vi "GUI_kHz_Control_Center_beta.vi"() -> ()   [LabVIEW 2020]
uses:
  GUI_TestStand/Fire button.ctl
  Shared/GUI_Template/GUI_master/tcp_new_data_event.ctl
  Shared/GUI_Template/GUI_master/tcp new data cluster.ctl
  Device Drivers/DG645/subVIs/TriggerSource_TypDef.ctl
panel:
  in  "BASE PATH":path=path "Z:/software/control-all-loasis/kHzLPA/Developers Version"
  in  "stop":bool
  in  "Tab Control":enum32{"Devices", "Parameters"}(tab)=enum."Parameters"
  in  "GUIdevice 6":string="kHz_Zaber_Compressor"
  in  "GUIdevice 2":string="kHz_1Wire"
  in  "GUIdevice 1":string="kHz_Alicat"
  in  "GUIdevice 3":string="kHz_Hexapod_Target"
  in  "GUIdevice 4":string="kHz_DG645_ShotControl"
  in  "GUIdevice 5":string="kHz_Zaber_Compressor"
  out "error IO":errorcluster
  out "tcp data event":T1
  in  "fire::4":string="fire>>force" caption="fire text"
  in  "Step size":dbl=0.01 min=0.001 max=1.0 step=0.001 format="%.3f"
  in  "Rate (Hz)":dbl=0.3
  in  "Allow Fire Continues":bool
  out "Fire continues Indicator":bool caption="Fire continuous"
  in  "Trigger.Source::4":T2 caption="SRS Trigger Mode"
  in  "LVStarter":bool caption="PicoL GUI"
  in  "Scan":T3(ring)
  in  "<command>::3":bool caption="ABORT"
  in  "Position.Ch1::5":i32 caption="Ch1" min=0 max=250000 step=1
  in  "Google Drive":bool
  in  "MasterControl":bool caption="PicoL GUI"
  in  "GEECSplot":bool caption="PicoL GUI"
  in  "AddColumns":bool caption="PicoL GUI"
  in  "DB Editor":bool caption="PicoL GUI"
  in  "Exp Editor":bool caption="PicoL GUI"
  in  "kHz Interactive":bool caption="PicoL GUI"
  in  "RemoteDesktop":bool caption="PicoL GUI"
  in  "Search Log":bool caption="PicoL GUI"
  in  "New Google\nExpLog for new day?":bool=TRUE
  in  "LogEpilog":bool caption="LogTable"
  in  "Create Log":bool caption="LogTable"
  in  "Position.Channel 1::2":T4(ring) caption="XH1"
  in  "Position.Channel 2::2":T4(ring) caption="XH2"
  in  "Position.Channel 3::2":T4(ring) caption="XH3"
  in  "Position.Channel 4::2":T4(ring) caption="XH4"
  in  "Position.Channel 5::2":T4(ring) caption="d-scan wedge"
  in  "Position.Channel 6::2":T4(ring) caption="EC wedge"
  in  "Position.Channel 8::2":T4(ring) caption="ND6+"
  in  "Position.Channel 7::2":T4(ring) caption="ExitMode wedge"
  in  "Pressure.device 1::1":dbl=3.6 caption="Target Pressure" min=0.0 max=100.0
  in  "Pressure.device 2::1":dbl=10.0 caption="Fiber Pressure" min=-14.7 max=300.0
  in  "xpos::3":dbl=-18.95 caption="x" min=-22.5 max=22.5 step=0.1 format="%.3f"
  in  "zpos::3":dbl=-0.7 caption="z" min=-10.0 max=10.0 step=0.1 format="%.3f"
  in  "ypos::3":dbl=10.7 caption="y" min=-22.5 max=22.5 step=0.1 format="%.3f"
  in  "uangle::3":dbl caption="u" min=-7.5 max=7.5 step=0.1 format="%.3f"
  in  "vangle::3":dbl=0.0007 caption="v" min=-7.5 max=7.5 step=0.1 format="%.3f"
  in  "wangle::3":dbl=-0.0001 caption="w" min=-7.5 max=7.5 step=0.1 format="%.3f"
  in  "LogTable":bool
  in  "Fire Button":T5=TRUE
  in  "Jet trigger":bool caption="Jet Trigger"
  in  "Jet enable":bool caption="Jet Enable"
  in  "Set opening time (s)":dbl=0.004
  in  "Amplitude.Ch AB::4":dbl=4.0 caption="Amplitude Jet trigger" min=0.5 max=5.0 format="%.1f"
  in  "Delay.Ch B::4":dbl=0.004 caption="Opening time" min=-0.1 max=0.1 format="%#_6p"
  in  "value0:6":bool caption="Fire continues"
  in  "UDP error message":string
  # "kHz Control Center"
  # "Laser"
  # "1-wire flippers"
  # "\"+x\" is towards laser table\n\"+y\" is towards OAP\n\"+z\" is up"
  # "ABORT !"
  # "Tobi's LogMaker"
  # "Alicat"
  # "New\nScan\nTable"
  # "Compressor"
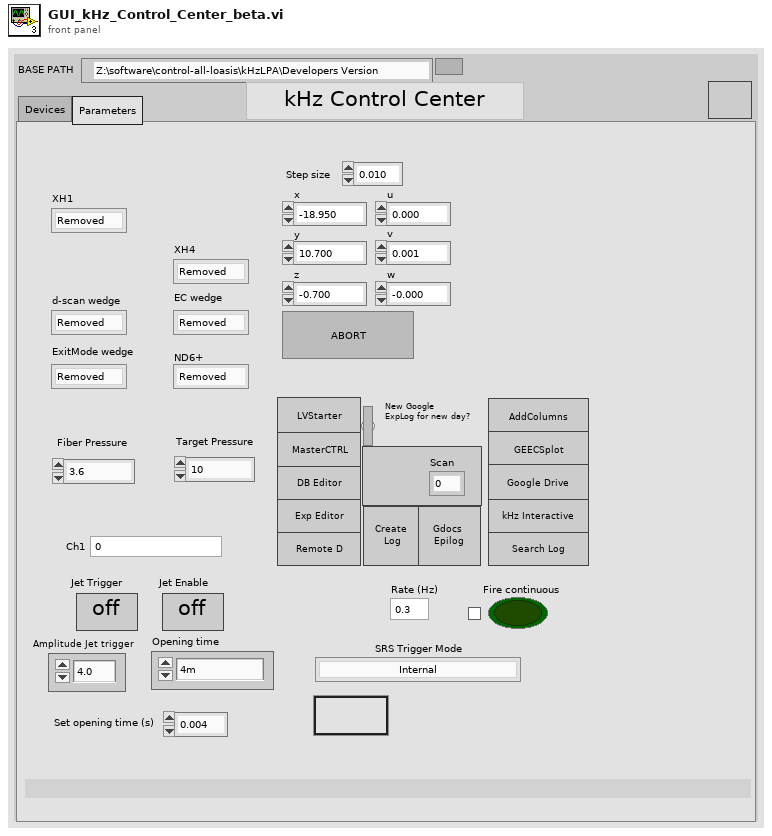
[diagram p1: front panel]
types:
  T1 = typedef "tcp_new_data_event.ctl" = refnum<user-event>
  T2 = typedef "TriggerSource_TypDef.ctl" = enum16{"Internal", "External rising edges", "External falling edges", "Single shot external rising edges", "Single shot external falling edges", "Single shot", "Line"}
  T3 = enum16{"0", "1", "2", "3", "4", "5", "6", "7", "8", "9", "10", "11", "12", "13", "14", "15", "16", "17", "18", "19", "20", "21", "22", "23", "24", "25", "26", "27", "28", "29", "30", "31", "32", "33", "34", "35", "36", "37", "38", "39", "40", "41", "42", "43", "44", "45", "46", "47", "48", "49", "50", "51", "52", "53", "54", "55", "56", "57", "58", "59", "60", "61", "62", "63", "64", "65", "66", "67", "68", "69", "70", "71", "72", "73", "74", "75", "76", "77", "78", "79", "81", "82", "83", "84", "85", "86", "87", "88", "89", "90", "91", "92", "93", "94", "95", "96", "97", "98", "99", ""}
  T4 = enum16{"Removed", "Inserted", "Unknown", "Moving"}
  T5 = typedef "Fire button.ctl" = bool
  T6 = typedef "tcp new data cluster.ctl" = cluster{"EventEnum":enum16{"new data", "connection status update"}, "Device name":string}
  T7 = enum32{"Invalid", "Standard", "Closed", "Hidden", "Minimized", "Maximized"}
  T8 = enum32{"invalid app kind", "Development System", "Run Time System", "Student Edition", "Embedded LabVIEW", "Evaluation", "Custom"}
  T9 = cluster{"Core":cluster{"Current VI Reference":refnum<vi>, "Close Panel on Exit?":bool}, "F":bool, "Jet trigger":bool, "Fire Continues Allowed":bool, "Tik1":u32}
  T10 = cluster{"Current VI Reference":refnum<vi>, "Close Panel on Exit?":bool}
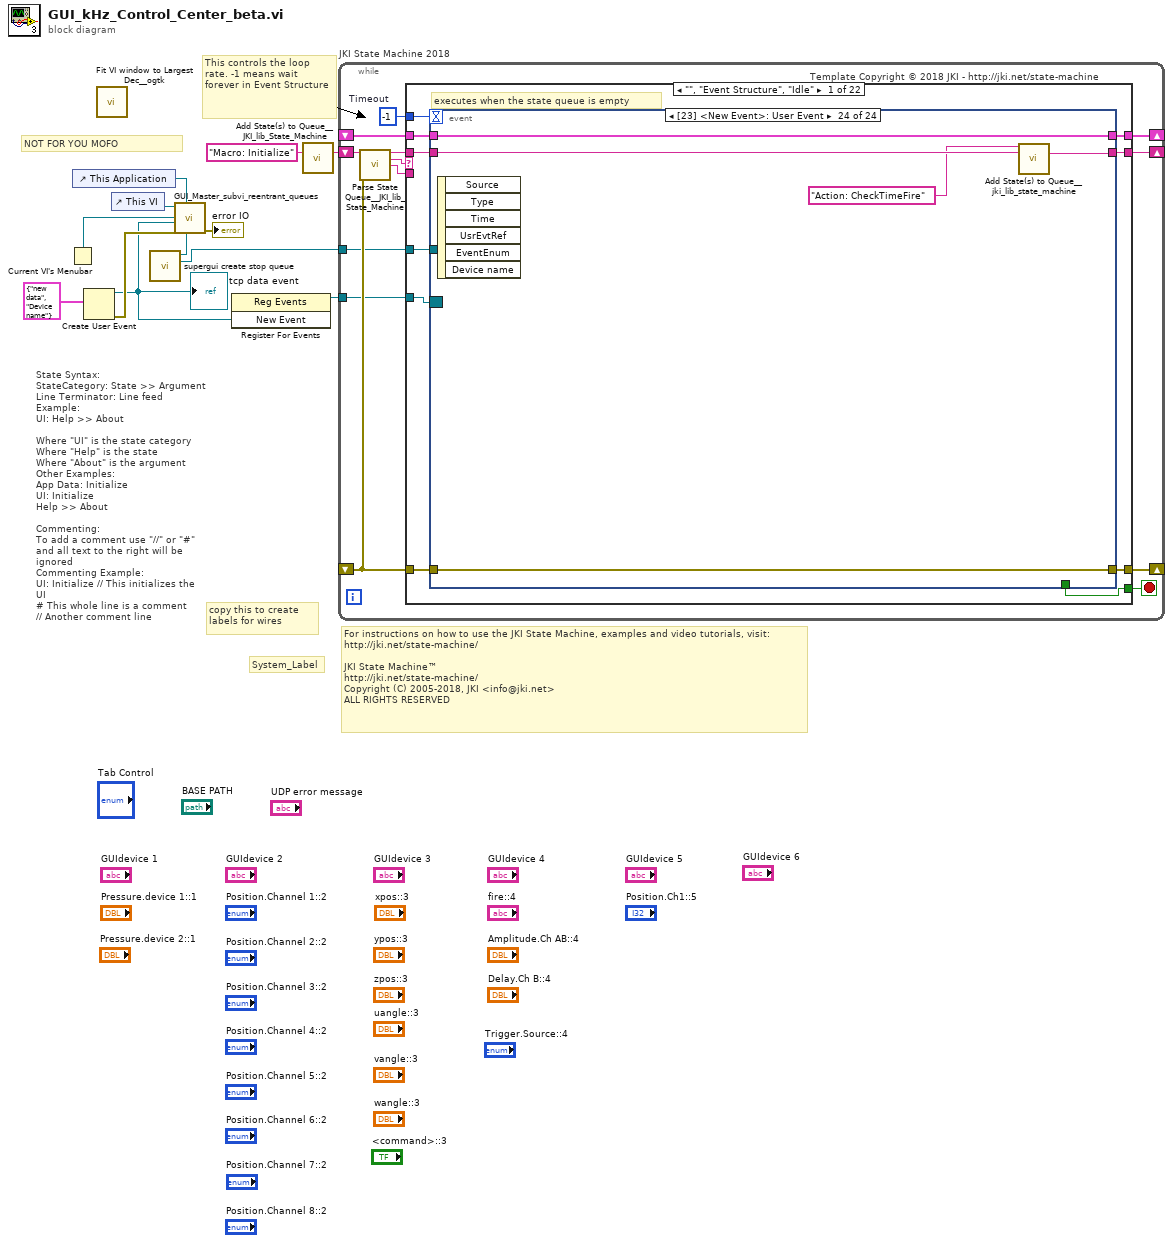
[diagram p0: block diagram]
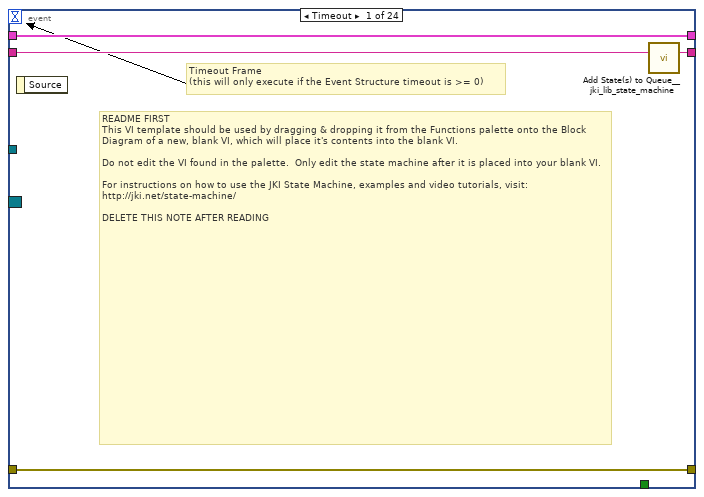
[diagram p2: hidden frame]
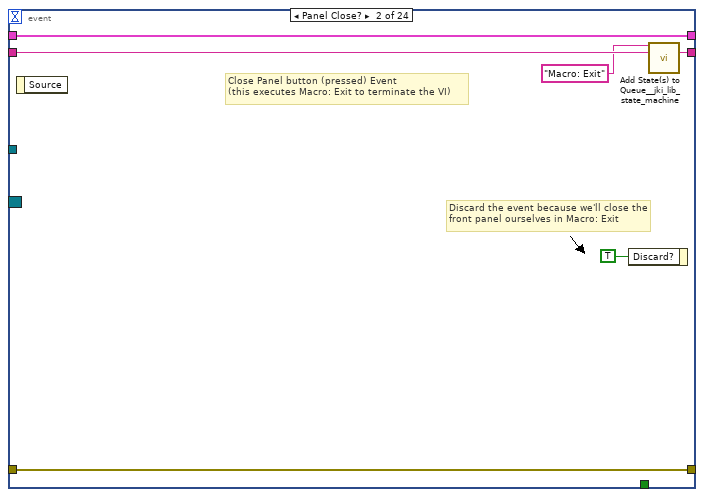
[diagram p3: hidden frame]
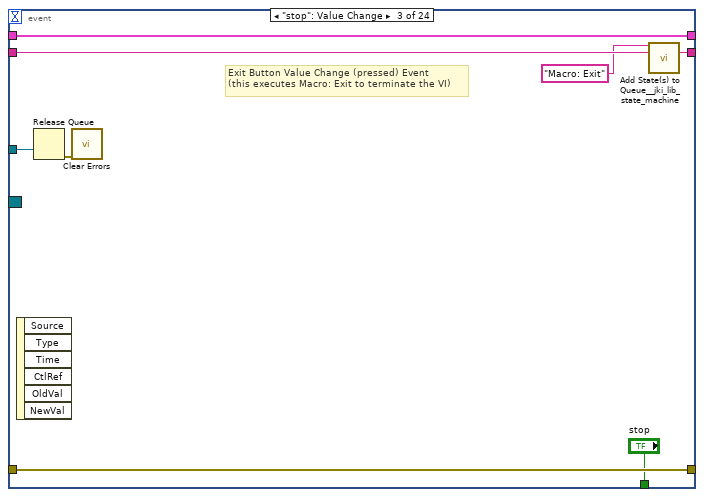
[diagram p4: hidden frame]
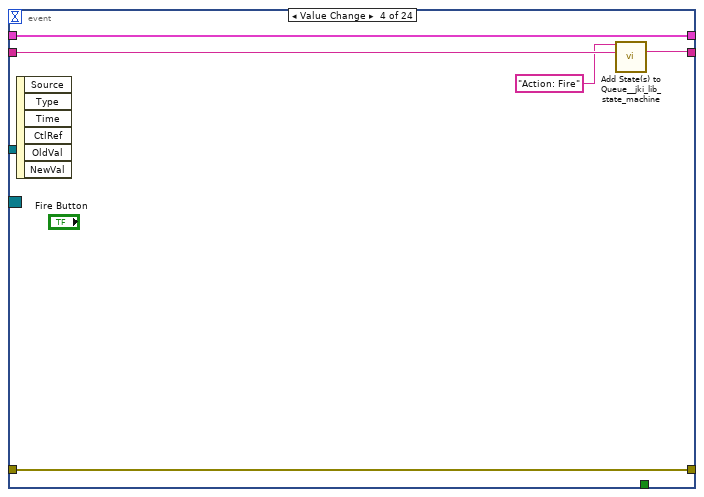
[diagram p5: hidden frame]
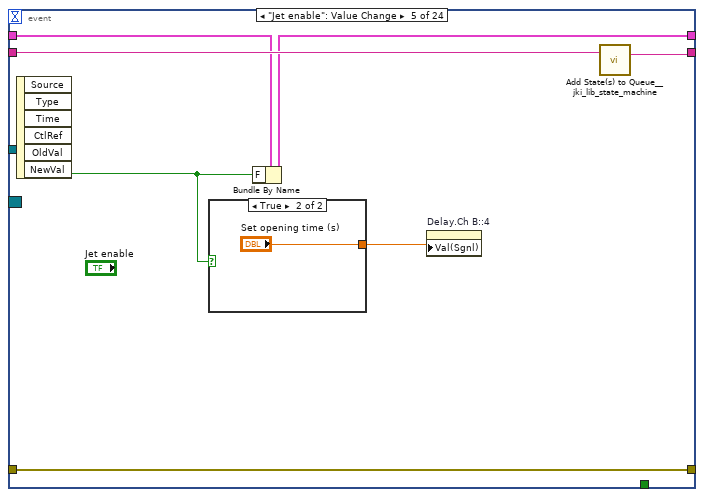
[diagram p6: hidden frame]
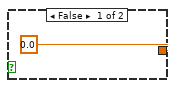
[diagram p7: hidden frame]
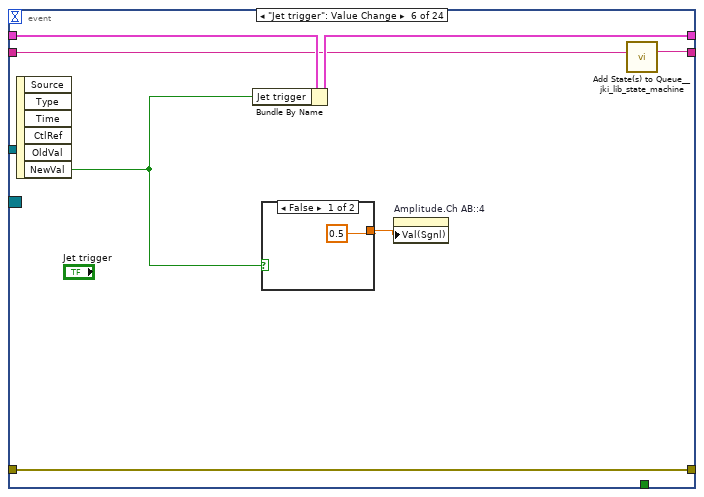
[diagram p8: hidden frame]
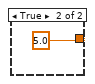
[diagram p9: hidden frame]
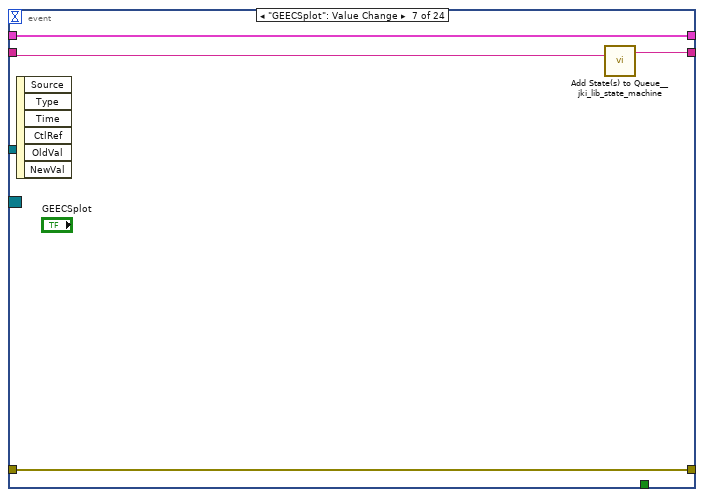
[diagram p10: hidden frame]
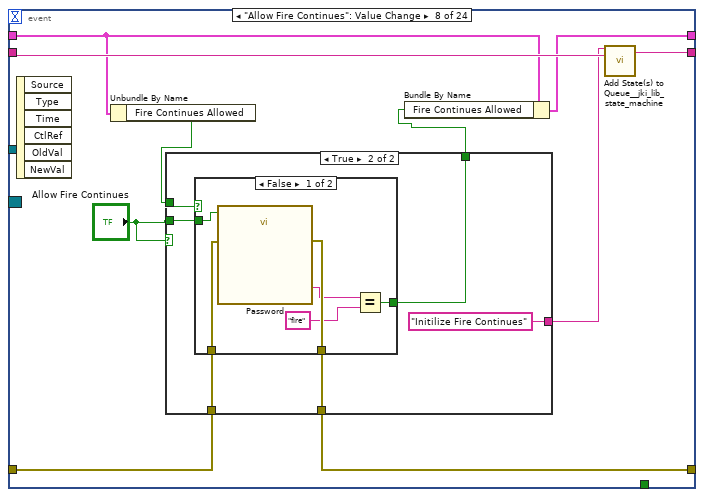
[diagram p11: hidden frame]
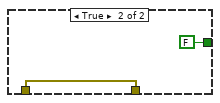
[diagram p13: hidden frame]
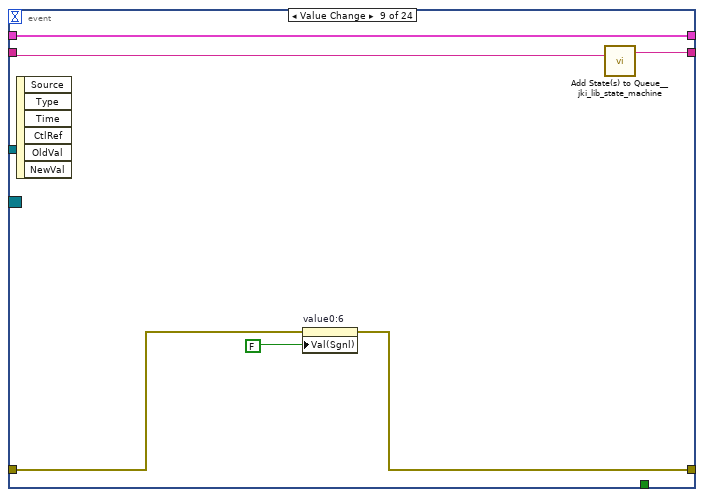
[diagram p14: hidden frame]
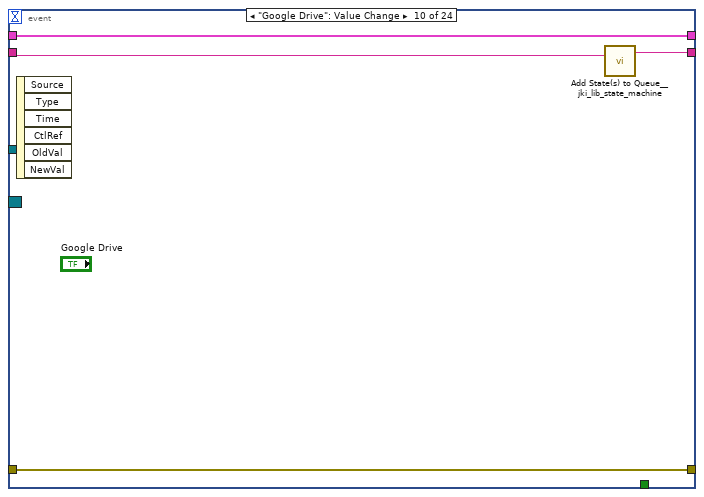
[diagram p15: hidden frame]
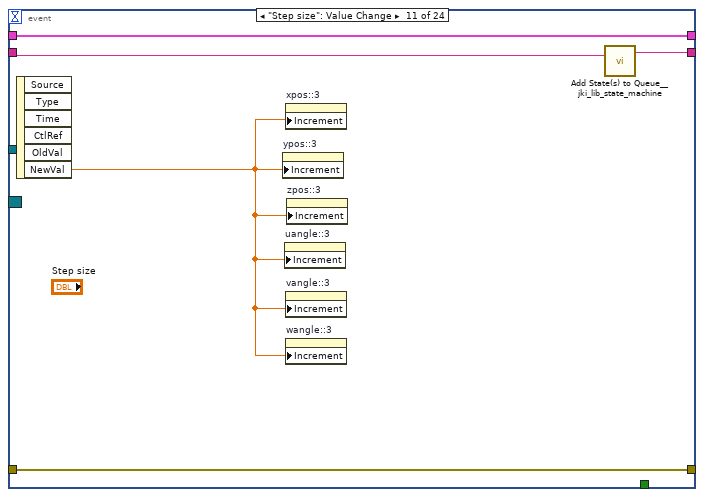
[diagram p16: hidden frame]
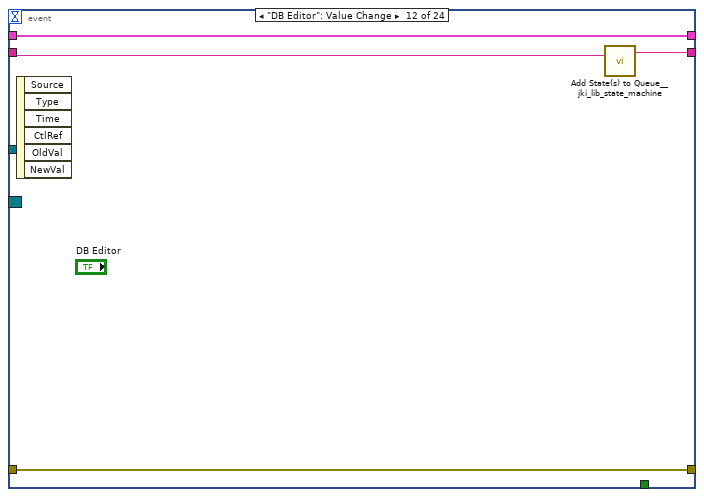
[diagram p17: hidden frame]
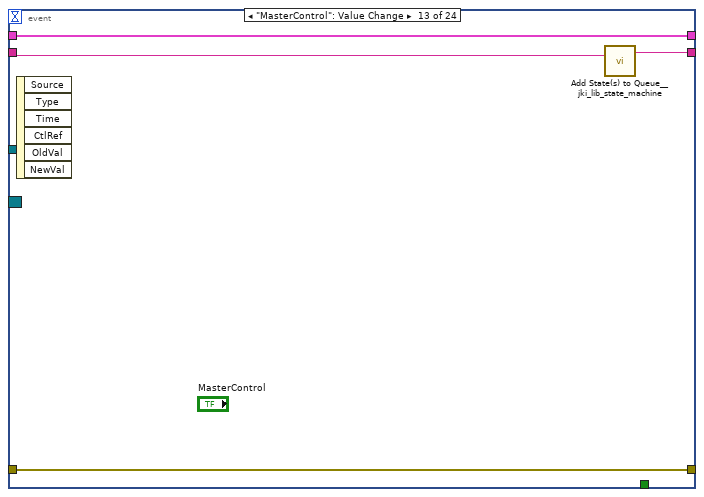
[diagram p18: hidden frame]
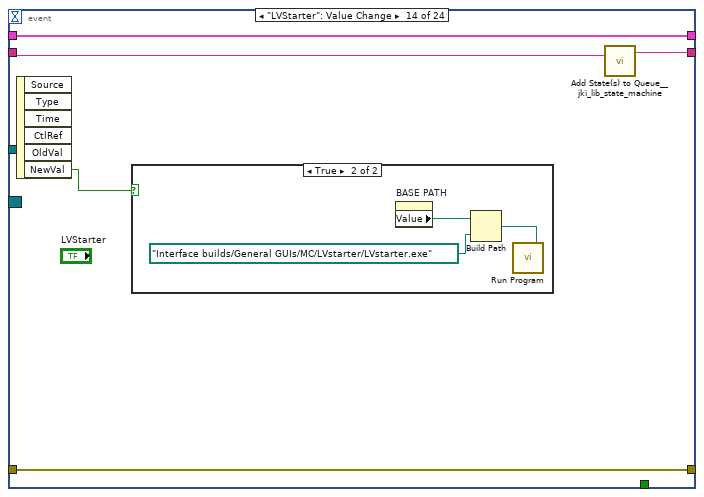
[diagram p19: hidden frame]
diagram:
  # "NOT FOR YOU MOFO"
  # "For instructions on how to use the JKI State Machine, examples and video tutorials, visit:\nhttp://jki.net/state-machine/\n\nJKI State Machine™\nhttp://jki.net/state-machine/\nCopyright (C) 2005-2018, JKI <info@jki.net>\nALL RIGHTS RESERVED"
  # "State Syntax:\nStateCategory: State >> Argument\nLine Terminator: Line feed\nExample:\nUI: Help >> About\n\nWhere \"UI\" is the state category\nWhere \"Help\" is the state\nWhere \"About\" is the argument\nOther Examples:\nApp Data: Initialize\nUI: Initialize\nHelp >> About\n\nCommenting:\nTo add a comment use \"//\" or \"#\" and all text to the right will be ignored\nCommenting Example:\nUI: Initialize // This initializes the UI\n# This whole line is a comment\n// Another comment line"
  # "copy this to create labels for wires"
  # "This controls the loop rate. -1 means wait forever in Event Structure"
  # "System_Label"
  n1 = Current VI's Menubar() -> (w6:refnum<k9>)
  n2 = control-ref of="This Application"() -> (w9:refnum<vi>)
  n3 = Create User Event(user event datatype=T6 {"EventEnum"=enum."new data", "Device name"="Device name"} ("New Event")) -> (user event=w3:refnum<user-event>, error out=w8:errorcluster)  [unwired: 1 in]
  "tcp data event" <- w3
  n4 = call <userlib>:"Fit VI window to Largest Dec__ogtk.vi"() -> ()  [unwired: 6 in, 2 out]
  n5 = control-ref of="This VI"() -> (w5:refnum<vi>)
  n6 = call "supergui create stop queue.vi"() -> ("STOP Queue out"=w2:refnum<queue>)  [unwired: 11 in]
  n7 = call "GUI_Master_subvi_reentrant_queues.vi"("STOP Queue in"=w2, "This Application"=w9, "error in (no error)"=w8, "tcp data event"=w3, "Caller menu reference"=w6, "Caller VI ref"=w5) -> ("error out"=→"error IO":errorcluster)  [unwired: 5 in]
  n8 = register-events(w3) -> (reference out=w1:refnum<event-registration>)  [unwired: 2 in, 1 out]
  n9 = call <vilib>:"Add State(s) to Queue__JKI_lib_State_Machine.vi"("State(s) in (\"\")"="Macro: Initialize") -> ("States Out"=w11:string)  [unwired: 14 in]
  n10 = while "JKI State Machine 2018" {
    shift-right: [w17] -> _
    shift-left: _ -> [w16]
    shift-right: [w20] -> _
    shift-left: _ -> [w14]
    shift-right: [w19] -> _
    shift-left: w11 -> [w21]
    tunnel: w2 -> [w13]
    tunnel: w1 -> [w12]
    stop <- w18 stop-if-true
    w15 = -1  # Timeout
    # "Template Copyright © 2018 JKI - http://jki.net/state-machine"
    n11 = call <vilib>:"Parse State Queue__JKI_lib_State_Machine.vi"("State Queue"=w21, "Error In (no error)"=w14) -> ("Remaining States"=w23:string, "Current State"=w24:string, "Arguments"=w22:string)  [unwired: 11 in]
    n12 = case shown="\"\", \"Event Structure\", \"Idle\"" w24 {
      selector: w24 -> [_ _ w182 _ _ _ _ _ _ _ _ _ _ _ _ _ _ _ _ _ _ _]
      tunnel: w23 -> [w34 w181 w186 w205 w211 w216 w220 w229 w235 w239 w243 w249 w260 w329 w334 w344 w348 w354 w358 w366 w378 w397]
      tunnel: w22 -> [_ _ _ _ _ _ _ _ _ _ _ w244 w254 _ _ _ _ _ _ _ _ _]
      tunnel: w16 -> [w32 w178 w184 w198 w208 w214 w217 _ w230 w236 w241 w247 w256 w326 w331 w341 w345 w352 w356 w361 w370 w382]
      tunnel: [w31 w179 w188 w202 errorcluster {"status"=FALSE, "code"=0, "source"=""} ("error out") w213 w218 w226 w231 w237 w240 w245 w257 w327 w332 w342 w346 w349 w355 w359 w368 w395] -> w20
      tunnel: w14 -> [w30 w179 w187 w202 w207 w213 w218 w226 w232 w237 w240 w246 w258 w327 w332 w342 w346 w350 w355 w360 w367 w395]
      tunnel: [w33 w180 w185 w204 w210 w215 w219 w228 w234 w238 w242 w248 w259 w328 w333 w343 w347 w353 w357 w365 w377 w396] -> w19
      tunnel: [w26 _ _ _ _ TRUE _ _ _ _ _ _ _ _ _ _ _ _ _ _ _ _] -> w18
      tunnel: [w29 w178 w184 w203 w208 w214 w217 w227 w230 w236 w241 w247 w256 w326 w331 w341 w345 w352 w356 w361 w369 w381] -> w17
      tunnel: w15 -> [w28 _ _ _ _ _ _ _ _ _ _ _ _ _ _ _ _ _ _ _ _ _]
      tunnel: w13 -> [w27 _ _ _ _ _ _ _ _ _ _ _ _ _ _ _ _ _ _ _ _ _]
      tunnel: w12 -> [w25 _ _ _ _ _ _ _ _ _ _ _ _ _ _ _ _ _ _ _ _ _]
      frame "", "Event Structure", "Idle" {
        # "executes when the state queue is empty"
        n13 = event shown="[23] <New Event>: User Event" {
          selector: w25 -> [_ _ _ _ _ _ _ _ _ _ _ _ _ _ _ _ _ _ _ _ _ _ _ _]
          dyn-events: _ -> [_ _ _ _ _ _ _ _ _ _ _ _ _ _ _ _ _ _ _ _ _ _ _ _]
          timeout: w28 -> [_ _ _ _ _ _ _ _ _ _ _ _ _ _ _ _ _ _ _ _ _ _ _ _]
          tunnel: w34 -> [w38 w44 w52 w56 w62 w67 w77 w88 w109 w113 w118 w122 w126 w130 w140 w144 w146 w150 w154 w158 w162 w166 w170 w175]
          tunnel: [w37 w43 w51 w57 w63 w68 w78 w89 w110 w114 w119 w123 w127 w131 w139 w143 w147 w151 w155 w159 w163 w167 w171 w176] -> w33
          tunnel: w32 -> [w35 w41 w49 w55 w61 w72 w79 w87 w111 w115 w120 w124 w128 w132 w137 w141 w145 w149 w153 w157 w161 w165 w169 w174]
          tunnel: [w36 w42 w50 w53 w58 w69 w76 w80 w106 w112 w117 w121 w125 w129 w138 w142 w148 w152 w156 w160 w164 w168 w172 w177] -> w31
          tunnel: w30 -> [w36 w42 w50 w53 w58 w69 w76 w81 w107 w112 w117 w121 w125 w129 w138 w142 w148 w152 w156 w160 w164 w168 w172 w177]
          tunnel: [w35 w41 w49 w55 w60 w70 w79 w86 w111 w115 w120 w124 w128 w132 w137 w141 w145 w149 w153 w157 w161 w165 w169 w174] -> w29
          tunnel: w27 -> [_ _ w46 _ _ _ _ _ _ _ _ _ _ _ _ _ _ _ _ _ _ _ _ _]
          tunnel: [_ _ "stop" _ _ _ _ _ _ _ _ _ _ _ _ _ _ _ _ _ _ _ _ _] -> w26
          event Timeout {
            # "README FIRST\nThis VI template should be used by dragging & dropping it from the Functions palette onto the Block Diagram of a new, blank VI, which will place it's contents into the blank VI.\n\nDo not edit the VI found in the palette.  Only edit the state machine after it is placed into your blank VI.\n\nFor instructions on how to use the JKI State Machine, examples and video tutorials, visit:\nhttp://jki.net/state-machine/\n\nDELETE THIS NOTE AFTER READING"
            # "Timeout Frame\n(this will only execute if the Event Structure timeout is >= 0)"
            n14 = event-data() -> ()  [unwired: 1 in, 1 out]
            n15 = call <vilib>:"Add State(s) to Queue__jki_lib_state_machine.vi"("State(s) in (\"\")"=w38) -> ("States Out"=w37:string)  [unwired: 14 in]
          }
          event Panel Close? {
            # "Discard the event because we'll close the front panel ourselves in Macro: Exit"
            # "Close Panel button (pressed) Event\n(this executes Macro: Exit to terminate the VI)"
            n16 = event-data() -> ()  [unwired: 1 in, 1 out]
            n17 = event-data("Discard?"=TRUE) -> ()  [unwired: 1 in, 1 out]
            n18 = call <vilib>:"Add State(s) to Queue__jki_lib_state_machine.vi"("State(s) in Front (\"\")"="Macro: Exit", "State(s) in (\"\")"=w44) -> ("States Out"=w43:string)  [unwired: 13 in]
          }
          event "stop": Value Change {
            # "Exit Button Value Change (pressed) Event\n(this executes Macro: Exit to terminate the VI)"
            n19 = event-data() -> ()  [unwired: 1 in, 6 out]
            n20 = Release Queue(queue=w46) -> (error out=w47:errorcluster)  [unwired: 2 in, 2 out]
            n21 = call <vilib>:"Clear Errors.vi"("error in (no error)"=w47) -> ()  [unwired: 5 in, 2 out]
            n22 = call <vilib>:"Add State(s) to Queue__jki_lib_state_machine.vi"("State(s) in Front (\"\")"="Macro: Exit", "State(s) in (\"\")"=w52) -> ("States Out"=w51:string)  [unwired: 13 in]
          }
          event Value Change {
            n23 = event-data() -> ()  [unwired: 1 in, 6 out]
            n24 = call <vilib>:"Add State(s) to Queue__jki_lib_state_machine.vi"("State(s) in Front (\"\")"="Action: Fire" ("State(s) in Front (\"\")"), "State(s) in (\"\")"=w56) -> ("States Out"=w57:string)  [unwired: 13 in]
          }
          event "Jet enable": Value Change {
            n25 = event-data() -> ("NewVal"=w59:bool)  [unwired: 1 in, 5 out]
            n26 = case shown="True" w59 {
              tunnel: [0.0 ("opening Time") "Set opening time (s)"] -> w64
              frame False {
              }
              frame True {
              }
            }
            n27 = Bundle By Name(cluster=w61, "F"=w59) -> (w60:T9)
            n28 = property on="Delay.Ch B::4" class="DigNum (strict)"("Val(Sgnl)"=w64) -> ()  [unwired: 2 in, 2 out]
            n29 = call <vilib>:"Add State(s) to Queue__jki_lib_state_machine.vi"("State(s) in (\"\")"=w62) -> ("States Out"=w63:string)  [unwired: 14 in]
          }
          event "Jet trigger": Value Change {
            n30 = event-data() -> ("NewVal"=w71:bool)  [unwired: 1 in, 5 out]
            n31 = Bundle By Name(cluster=w72, "Jet trigger"=w71) -> (w70:T9)
            n32 = case shown="False" w71 {
              tunnel: [0.5 ("Amplitude.Ch CD::10") 5.0 ("Amplitude.Ch CD::10")] -> w73
              frame False {
              }
              frame True {
              }
            }
            n33 = property on="Amplitude.Ch AB::4" class="DigNum (strict)"("Val(Sgnl)"=w73) -> ()  [unwired: 2 in, 2 out]
            n34 = call <vilib>:"Add State(s) to Queue__jki_lib_state_machine.vi"("State(s) in (\"\")"=w67) -> ("States Out"=w68:string)  [unwired: 14 in]
          }
          event "GEECSplot": Value Change {
            n35 = event-data() -> ()  [unwired: 1 in, 6 out]
            n36 = call <vilib>:"Add State(s) to Queue__jki_lib_state_machine.vi"("State(s) in (\"\")"=w77) -> ("States Out"=w78:string)  [unwired: 14 in]
          }
          event "Allow Fire Continues": Value Change {
            n37 = event-data() -> ()  [unwired: 1 in, 6 out]
            n38 = Unbundle By Name(w87) -> ("Fire Continues Allowed"=w82:bool)
            n39 = case shown="True" "Allow Fire Continues" {
              tunnel: [w90 w97] -> w80
              tunnel: "Allow Fire Continues" -> [_ w96]
              tunnel: w81 -> [w90 w95]
              tunnel: w82 -> [w91 w94]
              tunnel: [w91 w92] -> w84
              tunnel: [_ "Initilize Fire Continues" ("State(s) in Front (\"\")")] -> w85
              frame False {
              }
              frame True {
                n40 = case shown="False" w94 {
                  tunnel: [w103 w104] -> w97
                  tunnel: w96 -> [w102 _]
                  tunnel: w95 -> [w101 w104]
                  tunnel: [w98 FALSE] -> w92
                  frame False {
                    n41 = call "Password"("Enable"=w102, "error in (no error)"=w101) -> ("Password"=w100:string, "error out"=w103:errorcluster)  [unwired: 15 in, 1 out]
                    n42 = Equal?(x=w100, y="fire") -> (x = y?=w98:bool)
                  }
                  frame True {
                  }
                }
              }
            }
            n43 = Bundle By Name(cluster=w87, "Fire Continues Allowed"=w84) -> (w86:T9)
            n44 = call <vilib>:"Add State(s) to Queue__jki_lib_state_machine.vi"("State(s) in Front (\"\")"=w85, "State(s) in (\"\")"=w88) -> ("States Out"=w89:string)  [unwired: 13 in]
          }
          event Value Change {
            n45 = event-data() -> ()  [unwired: 1 in, 6 out]
            n46 = property on="value0:6" class="Bool (strict)"(error in=w107, "Val(Sgnl)"=FALSE) -> (error out=w106:errorcluster)  [unwired: 1 in, 1 out]
            n47 = call <vilib>:"Add State(s) to Queue__jki_lib_state_machine.vi"("State(s) in (\"\")"=w109) -> ("States Out"=w110:string)  [unwired: 14 in]
          }
          event "Google Drive": Value Change {
            n48 = event-data() -> ()  [unwired: 1 in, 6 out]
            n49 = call <vilib>:"Add State(s) to Queue__jki_lib_state_machine.vi"("State(s) in (\"\")"=w113) -> ("States Out"=w114:string)  [unwired: 14 in]
          }
          event "Step size": Value Change {
            n50 = event-data() -> ("NewVal"=w116:dbl)  [unwired: 1 in, 5 out]
            n51 = property on="ypos::3" class="DigNum (strict)"("Increment"=w116) -> ()  [unwired: 2 in, 2 out]
            n52 = property on="uangle::3" class="DigNum (strict)"("Increment"=w116) -> ()  [unwired: 2 in, 2 out]
            n53 = property on="xpos::3" class="DigNum (strict)"("Increment"=w116) -> ()  [unwired: 2 in, 2 out]
            n54 = property on="vangle::3" class="DigNum (strict)"("Increment"=w116) -> ()  [unwired: 2 in, 2 out]
            n55 = property on="wangle::3" class="DigNum (strict)"("Increment"=w116) -> ()  [unwired: 2 in, 2 out]
            n56 = property on="zpos::3" class="DigNum (strict)"("Increment"=w116) -> ()  [unwired: 2 in, 2 out]
            n57 = call <vilib>:"Add State(s) to Queue__jki_lib_state_machine.vi"("State(s) in (\"\")"=w118) -> ("States Out"=w119:string)  [unwired: 14 in]
          }
          event "DB Editor": Value Change {
            n58 = event-data() -> ()  [unwired: 1 in, 6 out]
            n59 = call <vilib>:"Add State(s) to Queue__jki_lib_state_machine.vi"("State(s) in (\"\")"=w122) -> ("States Out"=w123:string)  [unwired: 14 in]
          }
          event "MasterControl": Value Change {
            n60 = event-data() -> ()  [unwired: 1 in, 6 out]
            n61 = call <vilib>:"Add State(s) to Queue__jki_lib_state_machine.vi"("State(s) in (\"\")"=w126) -> ("States Out"=w127:string)  [unwired: 14 in]
          }
          event "LVStarter": Value Change {
            n62 = event-data() -> ("NewVal"=w133:bool)  [unwired: 1 in, 5 out]
            n63 = case shown="True" w133 {
              frame False {
              }
              frame True {
                n64 = property on="BASE PATH" class="Path"() -> ("Value"=w134:path)  [unwired: 2 in, 2 out]
                n65 = Build Path(base path=w134, name or relative path=path "Interface builds/General GUIs/MC/LVstarter/LVstarter.exe") -> (appended path=w136:path)
                n66 = call "Run Program.vi"("Program Path"=w136) -> ()  [unwired: 1 in]
              }
            }
            n67 = call <vilib>:"Add State(s) to Queue__jki_lib_state_machine.vi"("State(s) in (\"\")"=w130) -> ("States Out"=w131:string)  [unwired: 14 in]
          }
          event "kHz Interactive": Value Change {
            n68 = event-data() -> ()  [unwired: 1 in, 6 out]
            n69 = call <vilib>:"Add State(s) to Queue__jki_lib_state_machine.vi"("State(s) in (\"\")"=w140) -> ("States Out"=w139:string)  [unwired: 14 in]
          }
          event "RemoteDesktop": Value Change {
            n70 = event-data() -> ()  [unwired: 1 in, 6 out]
            n71 = call <vilib>:"Add State(s) to Queue__jki_lib_state_machine.vi"("State(s) in (\"\")"=w144) -> ("States Out"=w143:string)  [unwired: 14 in]
          }
          event "Exp Editor": Value Change {
            n72 = event-data() -> ()  [unwired: 1 in, 6 out]
            n73 = call <vilib>:"Add State(s) to Queue__jki_lib_state_machine.vi"("State(s) in (\"\")"=w146) -> ("States Out"=w147:string)  [unwired: 14 in]
          }
          event "New Google\nExpLog for new day?": Value Change {
            n74 = event-data() -> ()  [unwired: 1 in, 6 out]
            n75 = call <vilib>:"Add State(s) to Queue__jki_lib_state_machine.vi"("State(s) in (\"\")"=w150) -> ("States Out"=w151:string)  [unwired: 14 in]
          }
          event "LogEpilog": Value Change {
            n76 = event-data() -> ()  [unwired: 1 in, 6 out]
            n77 = call <vilib>:"Add State(s) to Queue__jki_lib_state_machine.vi"("State(s) in (\"\")"=w154) -> ("States Out"=w155:string)  [unwired: 14 in]
          }
          event "LogTable": Value Change {
            n78 = event-data() -> ()  [unwired: 1 in, 6 out]
            n79 = call <vilib>:"Add State(s) to Queue__jki_lib_state_machine.vi"("State(s) in (\"\")"=w158) -> ("States Out"=w159:string)  [unwired: 14 in]
          }
          event "Search Log": Value Change {
            n80 = event-data() -> ()  [unwired: 1 in, 6 out]
            n81 = call <vilib>:"Add State(s) to Queue__jki_lib_state_machine.vi"("State(s) in (\"\")"=w162) -> ("States Out"=w163:string)  [unwired: 14 in]
          }
          event "AddColumns": Value Change {
            n82 = event-data() -> ()  [unwired: 1 in, 6 out]
            n83 = call <vilib>:"Add State(s) to Queue__jki_lib_state_machine.vi"("State(s) in (\"\")"=w166) -> ("States Out"=w167:string)  [unwired: 14 in]
          }
          event "Create Log": Value Change {
            n84 = event-data() -> ()  [unwired: 1 in, 6 out]
            n85 = call <vilib>:"Add State(s) to Queue__jki_lib_state_machine.vi"("State(s) in (\"\")"=w170) -> ("States Out"=w171:string)  [unwired: 14 in]
          }
          event User Event {
            n86 = event-data() -> ()  [unwired: 1 in, 6 out]
            n87 = call <vilib>:"Add State(s) to Queue__jki_lib_state_machine.vi"("State(s) in Front (\"\")"="Action: CheckTimeFire" ("State(s) in Front (\"\")"), "State(s) in (\"\")"=w175) -> ("States Out"=w176:string)  [unwired: 13 in]
          }
        }
      }
      frame "---------- Core ----------" {
        # "Do not put any code in this frame.\n(it is a separator no-op)"
        n88 = call <vilib>:"Add State(s) to Queue__JKI_lib_State_Machine.vi"("State(s) in (\"\")"=w181) -> ("States Out"=w180:string)  [unwired: 14 in]
      }
      frame Default {
        w191 = 42 items=["No error", "Argument error", "Memory is full", "Out of zone", "End of file", "File already open", "Generic file I/O error", "File not found", "File permission error", "Disk is full", "Duplicate path", "Too many files open", "System feature not enabled", "Resource file not found", "Cannot add resource", "Resource not found", "Image not found", "Image memory error", "Pen does not exist", "Config type invalid", "Config token not found", "Config parse error", "Config memory error", "Bad external code format", "Bad external code offset", "External code not present", "Null window", "Destroy window error", "Null menu", "Print aborted", "Bad print record", "Print driver error", "Windows error during printing", "Memory error during printing", "Print dialog error", "Generic print error", "Invalid device refnum", "Device not found", "Device parameter error", "Device unit error", "Cannot open device", "Device call aborted", "Generic error", "Cancelled by user", "Object ID too low", "Object ID too high", "Object not in heap", "Unknown heap", "Unknown object (invalid DefProc)", "Unknown object (DefProc not in table)", "Message out of range", "Invalid (null) method", "Unknown message", "Manager call not supported", "Bad address", "Network operation in progress", "Network operation timed out", "Connection is busy", "Network attribute not supported", "Network error", "Address in use", "System out of memory", "Connection aborted", "Connection refused", "Not connected", "Already connected", "Connection closed", "Initialization error (interapplication manager)", "Bad occurrence", "Wait on unbound occurrence handler", "Occurrence queue overflow", "Datalog type conflict", "Unused", "Unrecognized type (interapplication manager)", "Memory corrupt", "Failed to make temporary DLL", "Old CIN version", "Drag socket not found", "Failed to load drop-object", "Failed to register OLE object", "Failed to release OLE object", "Format specifier type mismatch", "Unknown format specifier", "Too few format specifiers", "Too many format specifiers", "Scan failed", "Newer CIN version", "Error converting to variant", "Runtime menu error", "Password tampered", "Variant attribute not found", "Incompatible variant data type", "Event data is not available", "Event Store is not present", "Occurrence is not found", "Event Queue is not created", "Event info is not available", "Refnum passed is NULL", "Error retrieving Class GUID", "Error retrieving CoClass GUID", "Error retrieving TypeLib GUID.", "Bad built application magic bytes.", "Specific driver is different from the specific driver associated with the Logical Name.", "There is no session opened to the class driver.", "Max Error", "MAX - Error with config objects", "MAX - Error loading configuration", "MAX - Group not supported"]
        # "Current State"
        # "Do not delete, rename, or modify this frame.\n(this is used to capture unhandled states and typos)"
        # "Handle mistyped state name (developer tool)"
        n89 = Format Into String(format string="Software Exception: Unhandled State \"%s\"." ("message"), error in=w187, w182) -> (resulting string=w190:string, error out=w189:errorcluster)  [unwired: 1 in]
        n90 = call <vilib>:"Error Cluster From Error Code.vi"("show call chain? (False)"=TRUE, "error in (no error)"=w189, "error message (\"\")"=w190, "error code (0)"=w191) -> ("error out"=w188:errorcluster)  [unwired: 5 in]
        n91 = call <vilib>:"Add State(s) to Queue__JKI_lib_State_Machine.vi"("State(s) in (\"\")"=w186) -> ("States Out"=w185:string)  [unwired: 14 in]
      }
      frame "Initialize Core Data" {
        # "Do not delete, rename, or modify this frame.\n(this is used to determine panel behavior on exit)"
        # "originally closed?"
        # "exe?"
        # "If panel starts closed or is an EXE, then close it when we exit"
        n92 = property class="VI"() -> ("FP.State"=w195:T7)  [unwired: 2 in, 2 out]
        n93 = property class="App"() -> ("App.Kind"=w201:T8)  [unwired: 2 in, 2 out]
        n94 = control-ref of="Current VI Reference"() -> (w196:refnum<vi>)
        n95 = Equal?(x=w195, y=T7."Closed" ("Front Panel Window:State")) -> (x = y?=w193:bool)
        n96 = Equal?(x=w201, y=T8."Run Time System" ("Application:Kind")) -> (x = y?=w199:bool)
        n97 = Or(x=w193, y=w199) -> (x .or. y?=w197:bool)
        n98 = Bundle By Name(cluster=w198, "Core.Current VI Reference"=w196, "Core.Close Panel on Exit?"=w197) -> (w203:T9)
        n99 = call <vilib>:"Add State(s) to Queue__JKI_lib_State_Machine.vi"("State(s) in (\"\")"=w205) -> ("States Out"=w204:string)  [unwired: 14 in]
      }
      frame "Error Handler" {
        # "Unhandled Error -- Display it"
        # "Handle any errors here.\nYou can also output any states to clean-up after errors occur"
        # "Clear error"
        n100 = call <vilib>:"General Error Handler.vi"("error in (no error)"=w207) -> ()  [unwired: 10 in, 5 out]
        n101 = call <vilib>:"Add State(s) to Queue__JKI_lib_State_Machine.vi"("State(s) in Front (\"\")"="/* Post Error States", "State(s) in (\"\")"=w211) -> ("States Out"=w210:string)  [unwired: 13 in]
      }
      frame "Exit" {
        # "Do not put any code in this frame.\n(No errors that occur here will be handled.)"
        n102 = call <vilib>:"Add State(s) to Queue__JKI_lib_State_Machine.vi"("State(s) in (\"\")"=w216) -> ("States Out"=w215:string)  [unwired: 14 in]
      }
      frame "---------- Data ----------" {
        # "Do not put any code in this frame.\n(It is a separator no-op. You can make a copy of this frame to create a new Data frame)"
        n103 = call <vilib>:"Add State(s) to Queue__JKI_lib_State_Machine.vi"("State(s) in (\"\")"=w220) -> ("States Out"=w219:string)  [unwired: 14 in]
      }
      frame "Data: Initialize" {
        w222 = TRUE  # Fire Continues Allowed
        w221 = u32 0  # Tik1
        w224 = FALSE  # F
        w223 = FALSE  # Jet trigger
        w225 = T10 {"Current VI Reference"=refnum, "Close Panel on Exit?"=FALSE}  # Core
        # "do not delete - used by framework"
        # "Expand Bundle to add new data elements to shift register data."
        # "Add new data here."
        # "Data names and types of shift register data are defined by this bundle."
        # "Initialize the shift-register data, here.\n(data names are defined by what you wire into the bundle function)"
        n104 = Bundle("Core"=w225, "F"=w224, "Jet trigger"=w223, "Fire Continues Allowed"=w222, "Tik1"=w221) -> (w227:T9)  [unwired: 1 in]
        n105 = call <vilib>:"Add State(s) to Queue__JKI_lib_State_Machine.vi"("State(s) in (\"\")"=w229) -> ("States Out"=w228:string)  [unwired: 14 in]
      }
      frame "Data: Cleanup" {
        # "Cleanup any data and references, here.\n(this is called automatically, by the Macro: Exit)"
        n106 = Unbundle By Name(w230) -> ("Core.Current VI Reference"=w233:refnum<vi>)
        n107 = Close Reference(reference=w233, error in (no error)=w232) -> (error out=w231:errorcluster)
        n108 = call <vilib>:"Add State(s) to Queue__JKI_lib_State_Machine.vi"("State(s) in (\"\")"=w235) -> ("States Out"=w234:string)  [unwired: 14 in]
      }
      frame "---------- UI ----------" {
        # "Do not put any code in this frame.\n(It is a separator no-op. You can make a copy of this frame to create a new UI frame)"
        n109 = call <vilib>:"Add State(s) to Queue__JKI_lib_State_Machine.vi"("State(s) in (\"\")"=w239) -> ("States Out"=w238:string)  [unwired: 14 in]
      }
      frame "UI: Initialize" {
        # "Initialize the User Interface, here.\n(this is called automatically, by the Macro: Init)"
        n110 = call <vilib>:"Add State(s) to Queue__JKI_lib_State_Machine.vi"("State(s) in (\"\")"=w243) -> ("States Out"=w242:string)  [unwired: 14 in]
      }
      frame "UI: Cursor Set" {
        # "Argument"
        # "Set and Unset Cursor Busy.\n(Usage: \"UI: Cursor Set >> Busy|Idle\")"
        n111 = case shown="\"Idle\", Default" w244 {
          tunnel: w246 -> [w251 w253]
          tunnel: [w250 w252] -> w245
          frame "Idle", Default {
            n112 = call <vilib>:"Unset Busy.vi"("error in (no error)"=w251) -> ("error out"=w250:errorcluster)  [unwired: 10 in]
          }
          frame "Busy" {
            n113 = call <vilib>:"Set Busy.vi"("error in (no error)"=w253) -> ("error out"=w252:errorcluster)  [unwired: 9 in, 1 out]
          }
        }
        n114 = call <vilib>:"Add State(s) to Queue__JKI_lib_State_Machine.vi"("State(s) in (\"\")"=w249) -> ("States Out"=w248:string)  [unwired: 14 in]
      }
      frame "UI: Front Panel State" {
        # "Argument"
        # "Set Front Panel Open or Closed\n(Usage: \"UI: Front Panel State >> Open|Close\")"
        n115 = Unbundle By Name(w256) -> ("Core.Current VI Reference"=w255:refnum<vi>)
        n116 = case shown="\"Minimize\", \"Minimized\"" w254 {
          tunnel: w258 -> [w266 w281 w292 w305 w318]
          tunnel: [w268 w282 w294 w307 w320] -> w257
          tunnel: w255 -> [w267 w279 w293 w306 w319]
          frame "Open", "Standard", Default {
            w261 = T7."Standard" ("State")
            n117 = property class="VI"(reference=w267, error in=w266) -> (reference out=w264:refnum<vi>, error out=w265:errorcluster, "FP.State"=w263:T7)
            n118 = Not Equal?(x=w263, y=w261) -> (x != y?=w262:bool)
            n119 = case shown="True" w262 {
              tunnel: [w272 w274] -> w268
              tunnel: w265 -> [w271 w274]
              tunnel: w264 -> [w270 _]
              tunnel: w261 -> [w269 _]
              frame True {
                n120 = invoke class="VI" method="FP.Open"(reference=w270, error in=w271, "Activate"=TRUE, "State"=w269) -> (error out=w272:errorcluster)  [unwired: 1 in, 4 out]
              }
              frame False {
              }
            }
          }
          frame "Close", "Closed" {
            n121 = property class="VI"(reference=w279, error in=w281) -> (reference out=w278:refnum<vi>, error out=w280:errorcluster, "FP.State"=w276:T7)
            n122 = Not Equal?(x=w276, y=T7."Closed" ("Front Panel Window:State")) -> (x != y?=w275:bool)
            n123 = case shown="True" w275 {
              tunnel: [w283 w286] -> w282
              tunnel: w280 -> [w283 w285]
              tunnel: w278 -> [_ w284]
              frame False {
              }
              frame True {
                n124 = invoke class="VI" method="FP.Close"(reference=w284, error in=w285) -> (error out=w286:errorcluster)  [unwired: 1 in, 2 out]
              }
            }
          }
          frame "Hidden", "Hide" {
            w287 = T7."Hidden" ("State")
            n125 = property class="VI"(reference=w293, error in=w292) -> (reference out=w290:refnum<vi>, error out=w291:errorcluster, "FP.State"=w289:T7)
            n126 = Not Equal?(x=w289, y=w287) -> (x != y?=w288:bool)
            n127 = case shown="True" w288 {
              tunnel: [w298 w299] -> w294
              tunnel: w291 -> [w297 w299]
              tunnel: w290 -> [w296 _]
              tunnel: w287 -> [w295 _]
              frame True {
                n128 = invoke class="VI" method="FP.Open"(reference=w296, error in=w297, "State"=w295) -> (error out=w298:errorcluster)  [unwired: 2 in, 4 out]
              }
              frame False {
              }
            }
          }
          frame "Minimize", "Minimized" {
            w300 = T7."Minimized" ("State")
            n129 = property class="VI"(reference=w306, error in=w305) -> (reference out=w303:refnum<vi>, error out=w304:errorcluster, "FP.State"=w302:T7)
            n130 = Not Equal?(x=w302, y=w300) -> (x != y?=w301:bool)
            n131 = case shown="True" w301 {
              tunnel: [w311 w312] -> w307
              tunnel: w304 -> [w310 w312]
              tunnel: w303 -> [w309 _]
              tunnel: w300 -> [w308 _]
              frame True {
                n132 = invoke class="VI" method="FP.Open"(reference=w309, error in=w310, "State"=w308) -> (error out=w311:errorcluster)  [unwired: 2 in, 4 out]
              }
              frame False {
              }
            }
          }
          frame "Maximize", "Maximized" {
            w313 = T7."Maximized" ("State")
            n133 = property class="VI"(reference=w319, error in=w318) -> (reference out=w316:refnum<vi>, error out=w317:errorcluster, "FP.State"=w315:T7)
            n134 = Not Equal?(x=w315, y=w313) -> (x != y?=w314:bool)
            n135 = case shown="True" w314 {
              tunnel: [w324 w325] -> w320
              tunnel: w317 -> [w323 w325]
              tunnel: w316 -> [w322 _]
              tunnel: w313 -> [w321 _]
              frame True {
                n136 = invoke class="VI" method="FP.Open"(reference=w322, error in=w323, "State"=w321) -> (error out=w324:errorcluster)  [unwired: 2 in, 4 out]
              }
              frame False {
              }
            }
          }
        }
        n137 = call <vilib>:"Add State(s) to Queue__JKI_lib_State_Machine.vi"("State(s) in (\"\")"=w260) -> ("States Out"=w259:string)  [unwired: 14 in]
      }
      frame "---------- Macro ----------" {
        # "Do not put any code in this frame.\n(It is a separator no-op. You can make a copy of this frame to create a new Macro frame)"
        n138 = call <vilib>:"Add State(s) to Queue__JKI_lib_State_Machine.vi"("State(s) in (\"\")"=w329) -> ("States Out"=w328:string)  [unwired: 14 in]
      }
      frame "Macro: Initialize" {
        w330 = "Data: Initialize\nInitialize Core Data\nUI: Initialize\nUI: Front Panel State >> Open"  # Data: Initialize Initialize Core Data UI: Initialize UI: Front Panel State >> Open
        # "Initialization Macro\n(This is called once, when the VI starts)"
        n139 = call <vilib>:"Add State(s) to Queue__JKI_lib_State_Machine.vi"("State(s) in Front (\"\")"=w330, "State(s) in (\"\")"=w334) -> ("States Out"=w333:string)  [unwired: 13 in]
      }
      frame "Macro: Exit" {
        # "Exit Macro\n(This is called once, when the VI exits)"
        n140 = Unbundle By Name(w341) -> ("Core.Close Panel on Exit?"=w340:bool)
        n141 = Select(t="UI: Front Panel State >> Close", s=w340, f="") -> (s? t:f=w337:string)
        n142 = call <vilib>:"Add State(s) to Queue__JKI_lib_State_Machine.vi"("State(s) in (\"\")"=w337, "State(s) at Back (\"\")"="Data: Cleanup\nExit") -> ("States Out"=w335:string)  [unwired: 13 in]
        n143 = call <vilib>:"Add State(s) to Queue__JKI_lib_State_Machine.vi"("State(s) in Front (\"\")"=w335, "State(s) in (\"\")"=w344) -> ("States Out"=w343:string)  [unwired: 13 in]
      }
      frame "---------- Action ----------" {
        # "Template Separator\n(You can make a copy of, or modify, this frame)"
        n144 = call <vilib>:"Add State(s) to Queue__JKI_lib_State_Machine.vi"("State(s) in (\"\")"=w348) -> ("States Out"=w347:string)  [unwired: 14 in]
      }
      frame "Action: Fire" {
        n145 = property on="fire::4" class="Str"(error in=w350, "Val(Sgnl)"="fire>>force" ("Value (Signaling)")) -> (error out=w349:errorcluster)  [unwired: 1 in, 1 out]
        n146 = call <vilib>:"Add State(s) to Queue__JKI_lib_State_Machine.vi"("State(s) in (\"\")"=w354) -> ("States Out"=w353:string)  [unwired: 14 in]
      }
      frame "Action: template" {
        n147 = call <vilib>:"Add State(s) to Queue__JKI_lib_State_Machine.vi"("State(s) in (\"\")"=w358) -> ("States Out"=w357:string)  [unwired: 14 in]
      }
      frame "Initilize Fire Continues" {
        n148 = Unbundle By Name(w361) -> ("Fire Continues Allowed"=w363:bool)
        n149 = property on="value0:6" class="Bool (strict)"(error in=w360, "Visible"=w363) -> (error out=w364:errorcluster)  [unwired: 1 in, 1 out]
        n150 = Not(x=w363) -> (.not. x?=w362:bool)
        n151 = property on="Fire continues Indicator" class="Bool (strict)"(error in=w364, "Visible"=w362) -> (error out=w359:errorcluster)  [unwired: 1 in, 1 out]
        n152 = call <vilib>:"Add State(s) to Queue__JKI_lib_State_Machine.vi"("State(s) in (\"\")"=w366) -> ("States Out"=w365:string)  [unwired: 14 in]
      }
      frame "Action: Check if Fire continues cllowed" {
        # "Check if it is allowed computer"
        # "Template Separator\n(You can make a copy of, or modify, this frame)"
        n153 = String To IP() -> (0:w374:u32)  [unwired: 1 in]
        n154 = IP To String(1:TRUE ("dot notation? (F)"), 2:w374) -> (0:w375:string)
        n155 = Equal?(x=w375, y="192.168.7.228") -> (x = y?=w371:bool)
        n156 = Not(x=w371) -> (.not. x?=w372:bool)
        n157 = Bundle By Name(cluster=w370, "Fire Continues Allowed"=w371) -> (w369:T9)
        n158 = property on="Allow Fire Continues" class="Bool (strict)"(error in=w367, "Visible"=w372) -> (error out=w368:errorcluster)  [unwired: 1 in, 1 out]
        n159 = call <vilib>:"Add State(s) to Queue__JKI_lib_State_Machine.vi"("State(s) in (\"\")"=w378) -> ("States Out"=w377:string)  [unwired: 14 in]
      }
      frame "Action: CheckTimeFire" {
        # "Your code here.\n(You can make a copy of, or modify, this frame)"
        n160 = Unbundle By Name(w382) -> ("Tik1"=w388:u32)
        n161 = Tick Count (ms)() -> (millisecond timer value=w386:u32)
        n162 = Unbundle By Name(w382) -> ("Fire Continues Allowed"=w392:bool)
        n163 = Reciprocal(x="Rate (Hz)") -> (1/x=w393:dbl)
        n164 = Subtract(x=w386, y=w388) -> (x-y=w385:u32)
        n165 = Multiply(x=1000.0, y=w393) -> (x*y=w394:dbl)
        n166 = Greater?(x=w385, y=w394) -> (0:w389:bool)
        n167 = And(x=w389, y="value0:6") -> (x .and. y?=w390:bool)
        n168 = And(x=w392, y=w390) -> (x .and. y?=w391:bool)
        n169 = case shown="True" w391 {
          tunnel: w386 -> [_ w400]
          tunnel: [w398 w400] -> w387
          tunnel: w388 -> [w398 _]
          tunnel: [_ "Action: Fire" ("State(s) in Front (\"\")")] -> w383
          frame False {
          }
          frame True {
          }
        }
        n170 = Bundle By Name(cluster=w382, "Tik1"=w387) -> (w381:T9)
        n171 = call <vilib>:"Add State(s) to Queue__JKI_lib_State_Machine.vi"("State(s) in Front (\"\")"=w383, "State(s) in (\"\")"=w397) -> ("States Out"=w396:string)  [unwired: 13 in]
        "Fire continues Indicator" <- "value0:6"
      }
    }
  }
